vi "test_ParseSolutionFile_ActiveTargets.vi"() -> (3 "Pass?":bool)   [LabVIEW 2019, in "Tests.SolutionBuilder.lvlib"]
uses:
  Tests.SolutionBuilder.lvlib
  SolutionBuilder/SolutionBuilder.lvclass
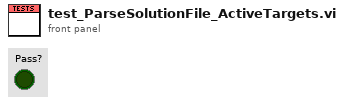
[diagram p1: front panel]
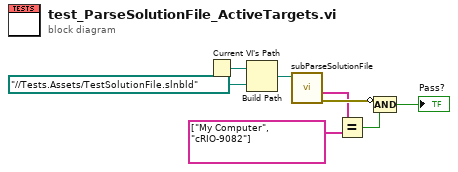
[diagram p0: block diagram]
diagram:
  n1 = Current VI's Path() -> (path=w7:path)
  n2 = Build Path(base path=w7, name or relative path=path "../../Tests.Assets/TestSolutionFile.slnbld" ("Path")) -> (appended path=w5:path)
  n3 = call "subParseSolutionFile.vi"("Solution file"=w5) -> ("error out"=w4:errorcluster, "Active targets"=w2:string[])  [unwired: 7 in, 2 out]
  n4 = Equal?(x=w2, y=string[] ["My Computer", "cRIO-9082"]) -> (x = y?=w3:bool)
  n5 = Compound Arithmetic op=AND(invert w4, w3) -> (→"Pass?":bool)
